vi "FilePath_Globals.vi"() -> ()   [LabVIEW 2020]
panel:
  in  "Calibrations Path":string="/home/lvuser/calibrations/"
  in  "Autonomous File Path":string="/home/lvuser/autonomous/"
  in  "Autonomous Paths File Path":string="/home/lvuser/autonomous/paths/"
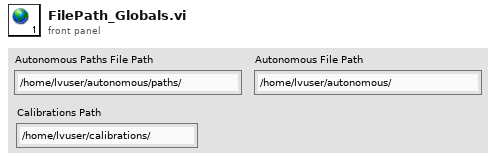
[diagram p1: front panel]
diagram:
